vi "LoadClass.vi"(0 "reference in":refnum<class "DAQ_Base.lvclass">, 1 "ClassName":string="NI_DAQ", 2 "LibBuildRootFolderName":string="DAQ_Module", 5 "error in (no error)":errorcluster) -> (14 "reference out":refnum<class "DAQ_Base.lvclass">, 19 "error out":errorcluster)   [LabVIEW 2020, in "DAQ.lvlib" / "DAQ_Base.lvclass"]
uses:
  DAQ_Base.lvclass
  <vilib>/addons/_AddQ/G#Object/G#Object.lvclass
panel:
  out "LibRootPath":path
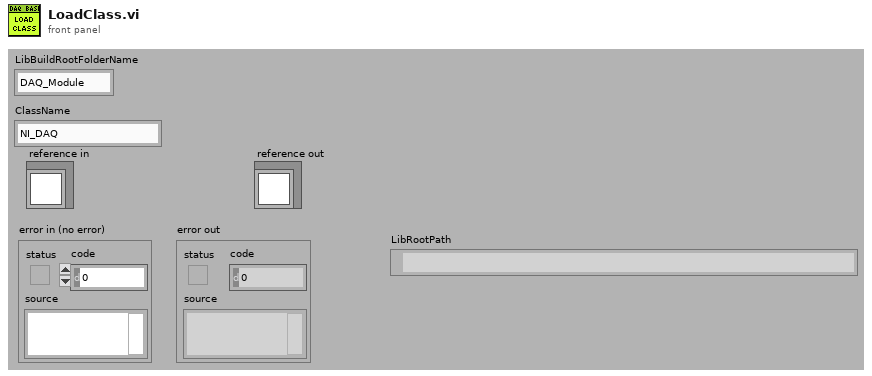
[diagram p1: front panel]
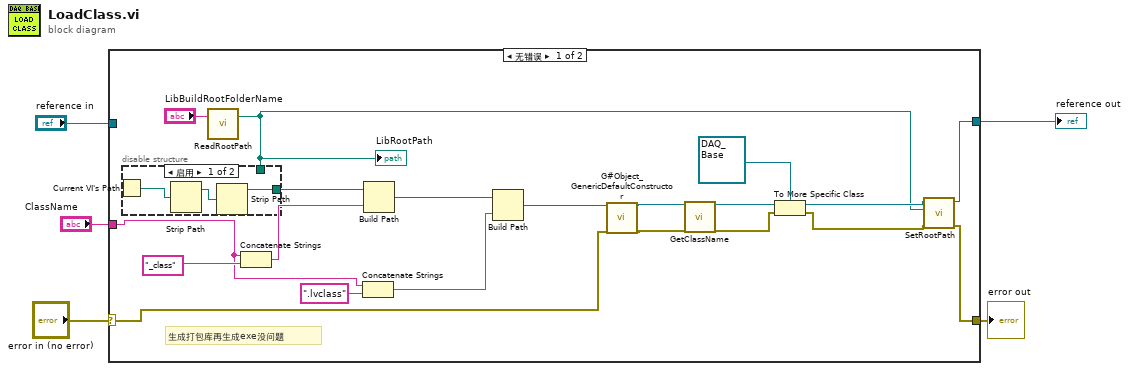
[diagram p0: block diagram]
diagram:
  n1 = case shown="无错误" "error in (no error)" {
    selector: "error in (no error)" -> [w13 w31]
    tunnel: [w9 w31] -> w4
    tunnel: "reference in" -> [_ w30]
    tunnel: "ClassName" -> [w14 _]
    tunnel: [w10 w30] -> w1
    frame No Error {
      # "生成打包库再生成exe没问题"
      n2 = call "ReadRootPath.vi"("LibBuildRootFolderName"="LibBuildRootFolderName") -> ("Root path"=w6:path)  [unwired: 18 in]
      "LibRootPath" <- w6
      n3 = disable-structure shown="启用" {
        disable-tunnel: [w28 w29] -> w25
        disable-tunnel: w6 -> [_ w29]
        frame Enabled {
          n4 = Current VI's Path() -> (path=w26:path)
          n5 = Strip Path(path=w26) -> (stripped path=w27:path)  [unwired: 1 out]
          n6 = Strip Path(path=w27) -> (stripped path=w28:path)  [unwired: 1 out]
        }
        frame Disabled {
        }
      }
      n7 = Concatenate Strings(w14, "_class" ("name or relative path")) -> (w21:string)
      n8 = Concatenate Strings "Concatenate Strings"(w14, ".lvclass" ("string")) -> (w18:string)
      n9 = Build Path(base path=w25, name or relative path=w21) -> (appended path=w17:path)
      n10 = Build Path(base path=w17, name or relative path=w18) -> (appended path=w22:path)
      n11 = call <vilib>:"G#Object_GenericDefaultConstructor.vi"("class path"=w22, "error in (no error)"=w13) -> ("reference out"=w23:refnum<class "G#Object.lvclass">, "error out"=w24:errorcluster)  [unwired: 15 in, 1 out]
      n12 = call-dynamic "GetClassName.vi"("reference in"=w23, "error in (no error)"=w24) -> ("reference out"=w16:refnum<class "G#Object.lvclass">, "error out"=w15:errorcluster)  [unwired: 13 in, 3 out]
      n13 = To More Specific Class(target class=refnum<class "DAQ_Base.lvclass"> refnum ("Base"), reference=w16, error in=w15) -> (specific class reference=w12:refnum<class "DAQ_Base.lvclass">, error out=w11:errorcluster)
      n14 = call-dynamic "SetRootPath.vi"("error in (no error)"=w11, "RootPath"=w6, "reference in"=w12) -> ("error out"=w9:errorcluster, "reference out"=w10:refnum<class "DAQ_Base.lvclass">)  [unwired: 7 in]
    }
    frame Error {
    }
  }
  "error out" <- w4
  "reference out" <- w1
